vi "RP100OperationComplete1.vi"() -> ()   [LabVIEW 2019, in "RP100.lvlib"]
uses:
  RP100.lvlib
panel:
  out "OperationComplete":dbl
  out "错误输出":errorcluster
  out "VISA资源名称输出":refnum<visa-resource-name>
  in  "错误输入（无错误）":errorcluster
  in  "VISA资源名称":refnum<visa-resource-name>
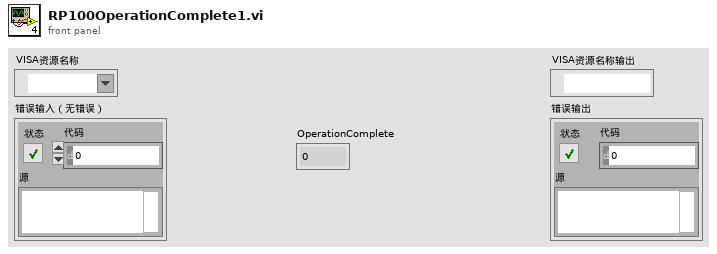
[diagram p1: front panel]
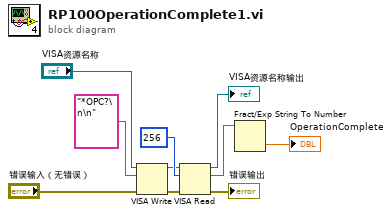
[diagram p0: block diagram]
diagram:
  n1 = VISA Write(VISA resource name="VISA资源名称", write buffer="*OPC?\n\n" ("写入缓冲区"), error in (no error)="错误输入（无错误）") -> (VISA resource name out=w4:refnum<visa-resource-name>, error out=w3:errorcluster)  [unwired: 1 out]
  n2 = VISA Read(VISA resource name=w4, byte count=u32 256 ("字节总数"), error in (no error)=w3) -> (VISA resource name out=→"VISA资源名称输出":refnum<visa-resource-name>, read buffer=w6:string, error out=→"错误输出":errorcluster)  [unwired: 1 out]
  n3 = Fract/Exp String To Number(string=w6) -> (number=→"OperationComplete":dbl)  [unwired: 3 in, 1 out]
